vi "_LO_GUNN_SET.vi"(8 "ATT":dbl, 9 "LO_ATT":u16(ring) items=["NEL VG", "Submm Beam", "WCA VD", "WG ATT"], 10 "Set@\nGunn Freq":dbl, 11 "Bias_LO_equip":T1={"Node address"=19, "CAN Interface"="CAN0", "Cartridge band"=10, "Slave Node in"={"Address"=19, "Serial Number"=[16, 71, 55, 76, 1, 8, 0, -15]}, "ObjHandle out"=159055936, "POL"=1, "sb"=1, "GPIB_SM (SIS S,V)"="24", "GPIB_DMM (SIS I)"="22", "GPIB_SM (MAG I) "="25", "GPIB_SG(LO)"="19", "GPIB_PW (PAMP) "="6", "GPIB_TMP1(8ch)"="12", "GPIB_TMP2(2ch)  "="13", "WCA_avg"=10, "Rsen"=10.0, "BiasModule"=1, "LOModule "=1, "WCA_LO_FREQ_SET"={"YTO Low freq. [GHz]"=14.42, "YTO High freq. [GHz]"=17.7, "Kvco"=1, "Lock Pol."=0, "SET LO FREQ"=72.5, "Multiplier"=6.0, "YTO (HEX)"=0, "YTO coarse( FREQ)"=25.0, "NULL PLL INTEGRATOR"=FALSE}, "Res for"=0} {"Res for" items=["none", "series res", "parallel res"]; "WCA_LO_FREQ_SET"."YTO coarse( FREQ)" min=25 max=150 step=0.0001 format="%.3f"; "WCA_LO_FREQ_SET"."Multiplier" min=3 max=6 step=3; "WCA_LO_FREQ_SET"."SET LO FREQ" min=25 max=150 step=0.0001 format="%.3f"; "WCA_LO_FREQ_SET"."Lock Pol." items=["Lower", "Upper"]; "WCA_LO_FREQ_SET"."Kvco" items=["7.5MHz/V", "15MHz/V"]; "WCA_LO_FREQ_SET"."YTO High freq. [GHz]" format="%.3f"; "WCA_LO_FREQ_SET"."YTO Low freq. [GHz]" format="%.3f"; "BiasModule" items=["B10Lab Bias", "WCA BiasModule"]; "Slave Node in"."Serial Number" format="%.0x"; "Slave Node in"."Address" format="%.0x"; "Cartridge band" max=10 step=1; "Node address" format="%.0x"}) -> ()   [LabVIEW 2017]
panel:
  out "Current":dbl(slide) scale=0.0..300.0
  out "Volt":dbl
  in  "GunnSet":bool
  # "LO freq. [GHz]"
  # "YTO LOW\n/High Freq."
  # "ZERO Intgrtr"
  # "Node Address"
  # "Serial Number"
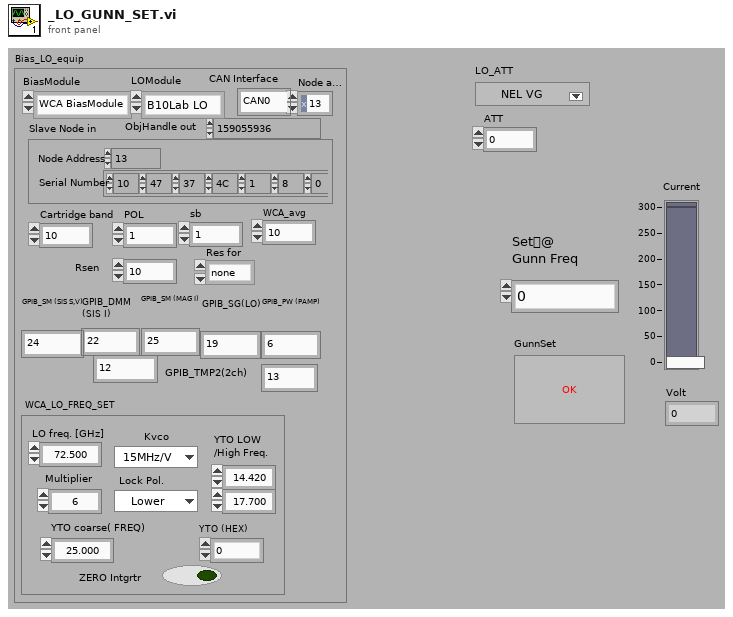
[diagram p1: front panel]
types:
  T1 = cluster{"Node address":u16, "CAN Interface":string, "Cartridge band":u32, "Slave Node in":cluster{"Address":i16, "Serial Number":i8[]}, "ObjHandle out":u32, "POL":u32, "sb":u32, "GPIB_SM (SIS S,V)":string, "GPIB_DMM (SIS I)":string, "GPIB_SM (MAG I) ":string, "GPIB_SG(LO)":string, "GPIB_PW (PAMP) ":string, "GPIB_TMP1(8ch)":string, "GPIB_TMP2(2ch)  ":string, "WCA_avg":i32, "Rsen":dbl, "BiasModule":u16, "LOModule ":u16, "WCA_LO_FREQ_SET":cluster{"YTO Low freq. [GHz]":sgl, "YTO High freq. [GHz]":sgl, "Kvco":u16, "Lock Pol.":u16, "SET LO FREQ":sgl, "Multiplier":sgl, "YTO (HEX)":u16, "YTO coarse( FREQ)":sgl, "NULL PLL INTEGRATOR":bool}, "Res for":u16}
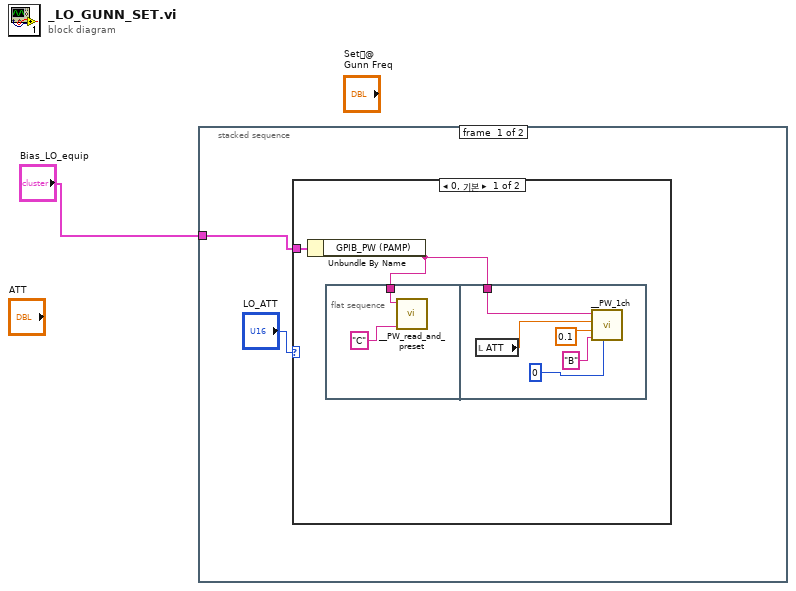
[diagram p0: block diagram]
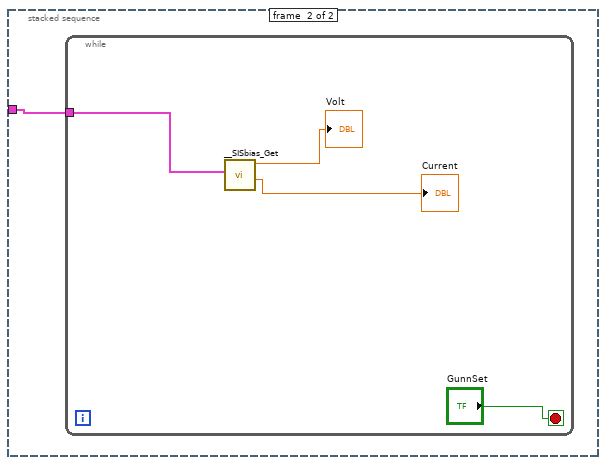
[diagram p3: hidden frame]
diagram:
  n1 = stacked-sequence {
    tunnel: "Bias_LO_equip" -> [w2 w13]
    frame #0 {
      n2 = case shown="0, 기본" "LO_ATT" {
        tunnel: w2 -> [w5 _]
        frame 0, Default {
          n3 = Unbundle By Name(w5) -> ("GPIB_PW (PAMP)"=w4:string)
          n4 = flat-sequence {
            tunnel: w4 -> [w6]
            tunnel: w4 -> [w10]
            frame #0 {
              n5 = call "__PW_read_and_preset.vi"("MAXChiA,B,C,Dj"="C", "GPIB"=w6) -> ()  [unwired: 10 in]
            }
            frame #1 {
              n6 = local read "ATT"() -> (w9:dbl)
              n7 = call "__PW_1ch.vi"("Wait(ms)"=0, "ChiA,B,C,Dj"="B", "A(A)"=0.1, "V(V)"=w9, "GPIB"=w10) -> ()  [unwired: 5 in, 2 out]
            }
          }
        }
        frame 1 {
        }
      }
    }
    frame #1 {
      n8 = while {
        tunnel: w13 -> [w16]
        stop <- "GunnSet" stop-if-true
        n9 = call "__SISbias_Get.vi"("Bias_LO_equip"=w16) -> ("Get_I(uA)"=→"Current":dbl, "Get_V(mV)"=→"Volt":dbl)  [unwired: 8 in, 1 out]
      }
    }
  }
